vi "PH_Stepmotor_BaseClass.Axis DIM open Services.vi"(0 "Instancename":string, 1 "Axis Number":i32, 2 "Axis Settings":T2, 5 "error in (no error)":errorcluster) -> (16 "Axis DIM Service IDs":T1, 19 "error out":errorcluster)   [LabVIEW 2014, in "PH_Stepmotor_BaseClass.lvlib"]
doc: "This VI opens several DIM services for a motion axis."
uses:
  PH_Stepmotor_BaseClass.lvlib
  PH_Stepmotor_BaseClass.Axis Settings.ctl
  PH_Stepmotor_BaseClass.Motor Type.ctl
  PH_Stepmotor_BaseClass.Axis DIM Service IDs.ctl
  PH_Stepmotor_BaseClass.Axis DIM Tags.ctl
  PH_Stepmotor_BaseClass.Axis Information.ctl
  PH_Stepmotor_BaseClass.Axis Activity.ctl
  PH_Stepmotor_BaseClass.Axis Address.ctl
  CSlibraries-extern/DimLVEvent/LVDimInterface/LVDimInterface.lvlib
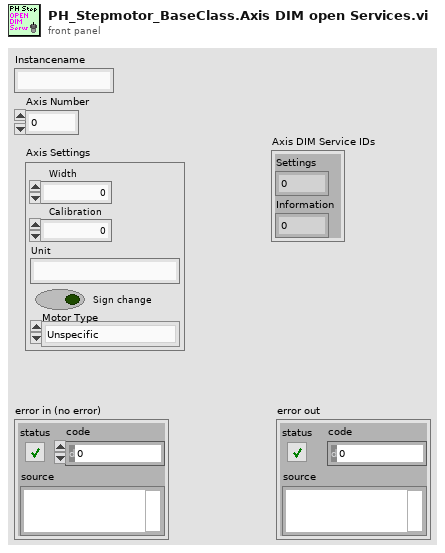
[diagram p1: front panel]
types:
  T1 = typedef "PH_Stepmotor_BaseClass.lvlib/PH_Stepmotor_BaseClass.Axis DIM Service IDs.ctl" = cluster{"Settings":i32, "Information":i32}
  T2 = typedef "PH_Stepmotor_BaseClass.lvlib/PH_Stepmotor_BaseClass.Axis Settings.ctl" = cluster{"Sign change":bool, "Width":dbl, "Calibration":dbl, "Unit":string, "Motor Type":T3, "Unit Width":string, "Unit CF":string}
  T3 = typedef "PH_Stepmotor_BaseClass.lvlib/PH_Stepmotor_BaseClass.Motor Type.ctl" = enum16{"Unspecific", "OWIS 49.120.2633", "OWIS 49.060.1033", "OWIS 43.040.2558", "Diamond Motion 2200 series", "OWIS 49.120.266B.MV6", "Calorimeter", "Linear Stage 1", "MICOS VT-80", "MICOS VT-80 S", "Standa Rotstage nt0.95A", "PUF RA 320.200", "PUF RA 800.200", "PUF RA 800.400", "PUF RA 400.50", "1324.nn.800.50", "1324.n9c.800.50", "1324.nn.320.200", "1324.nn.400.200", "1324.nn.800.200", "1324.nn.400.50", "1324.8c9c.800.50", "1324.8c9c.400.200"}
  T4 = typedef "PH_Stepmotor_BaseClass.lvlib/PH_Stepmotor_BaseClass.Axis Address.ctl" = cluster{"Instance":string, "Motor Nr":i32}
  T5 = typedef "PH_Stepmotor_BaseClass.lvlib/PH_Stepmotor_BaseClass.Axis Information.ctl" = cluster{"Scaled Position":dbl, "Activity":T6}
  T6 = typedef "PH_Stepmotor_BaseClass.lvlib/PH_Stepmotor_BaseClass.Axis Activity.ctl" = enum16{"No Information", "stopped", "running", "Failure", "Alarm", "stopped at backward ES", "stopped at foreward ES"}
  T7 = typedef "PH_Stepmotor_BaseClass.lvlib/PH_Stepmotor_BaseClass.Axis DIM Tags.ctl" = enum16{"no Info", "Information", "Settings"}
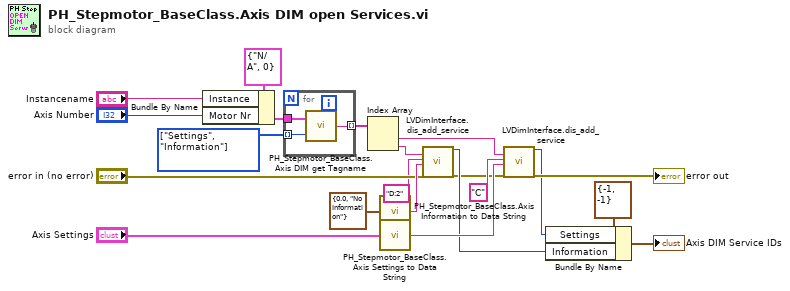
[diagram p0: block diagram]
diagram:
  w21 = T7[] [enum."Settings", enum."Information"] items=["no Info", "Information", "Settings"]
  n1 = Bundle By Name(cluster=T4 {"Instance"="N/A", "Motor Nr"=0} ("Address"), "Instance"="Instancename", "Motor Nr"="Axis Number") -> (w3:T4)
  n2 = for {
    tunnel: w3 -> [w24]
    tunnel: [w23] -> w18 mode=indexing
    tunnel: w21 -> [w22] mode=indexing
    n3 = call "PH_Stepmotor_BaseClass.Axis DIM get Tagname.vi"("Tag"=w22, "Instancename"=w24) -> ("Axis Tagname"=w23:string)
  }
  n4 = Index Array(array=w18) -> (element #1=w19:string, element #2=w1:string)  [unwired: 2 in]
  n5 = call "PH_Stepmotor_BaseClass.Axis Information to Data String.vi"("Axis Information"=T5 {"Scaled Position"=0.0, "Activity"=enum."No Information"}) -> ("Data String"=w17:string)
  n6 = call "PH_Stepmotor_BaseClass.Axis Settings to Data String.vi"("Axis Settings"="Axis Settings") -> ("Data String"=w16:string)
  n7 = call "LVDimInterface.dis_add_service.vi"("serviceName"=w1, "typeDescriptor"="D:2" ("data"), "data"=w17, "error in (no error)"="error in (no error)") -> ("my_serviceID"=w8:i32, "error out"=w2:errorcluster)  [unwired: 14 in]
  n8 = call "LVDimInterface.dis_add_service.vi"("serviceName"=w19, "typeDescriptor"="C" ("data"), "data"=w16, "error in (no error)"=w2) -> ("my_serviceID"=w9:i32, "error out"=→"error out":errorcluster)  [unwired: 14 in]
  n9 = Bundle By Name(cluster=T1 {"Settings"=-1, "Information"=-1} ("my_serviceID 3"), "Settings"=w9, "Information"=w8) -> (→"Axis DIM Service IDs":T1)
